vi "TRIGGER-completoN (SubVI).vi"(1 "Modalità":bool, 2 "isteresi":dbl, 3 "livello":dbl, 4 "Segnale B":dbl[](array[numeric])) -> (0 "eventi di trigger":i32[](array[numeric]))   [LabVIEW 2018]
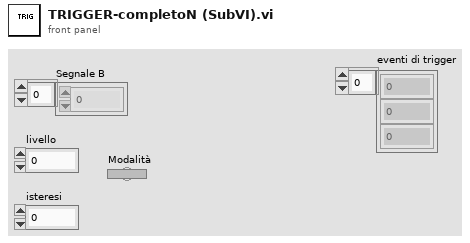
[diagram p1: front panel]
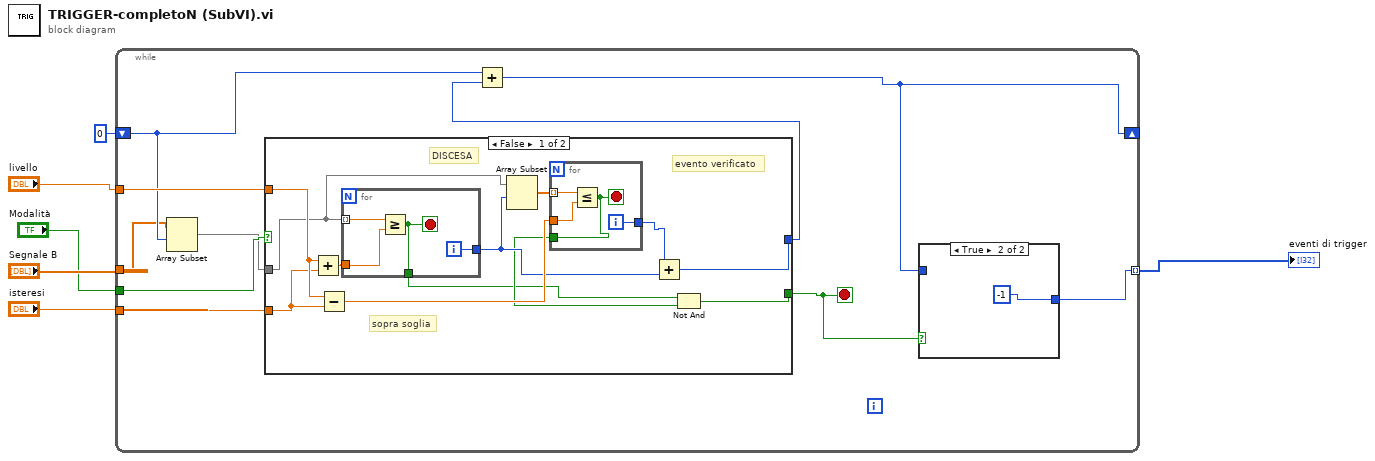
[diagram p0: block diagram]
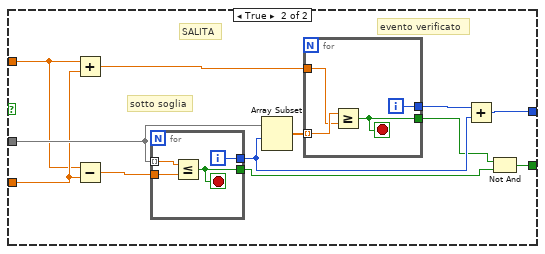
[diagram p3: hidden frame]
diagram:
  n1 = while {
    tunnel: "Segnale B" -> [w9]
    tunnel: "isteresi" -> [w16]
    tunnel: "livello" -> [w15]
    tunnel: [w11] -> w1 mode=indexing
    shift-right: [w8] -> _
    shift-left: 0 -> [w13]
    tunnel: "Modalità" -> [w12]
    stop <- w7 stop-if-true
    n2 = Array Subset(array=w9, index=w13) -> (w10:dbl[])  [unwired: 1 in]
    n3 = case shown="False" w12 {
      tunnel: w10 -> [w22 w49]
      tunnel: w16 -> [w24 w46]
      tunnel: w15 -> [w25 w45]
      tunnel: [w27 w42] -> w14
      tunnel: [w19 w41] -> w7
      frame False {
        # "evento verificato"
        # "sopra soglia"
        # "DISCESA"
        n4 = Add(x=w25, y=w24) -> (x+y=w26:dbl)
        n5 = Subtract(x=w25, y=w24) -> (x-y=w30:dbl)
        n6 = for {
          tunnel: [w38] -> w28
          tunnel: [w37] -> w20
          tunnel: w22 -> [w36] mode=indexing
          tunnel: w26 -> [w35]
          i -> [w38]
          stop <- w37 stop-if-true
          n7 = Greater Or Equal?(x=w36, y=w35) -> (x >= y?=w37:bool)
        }
        n8 = Array Subset(array=w22, index=w28) -> (w23:dbl[])  [unwired: 1 in]
        n9 = for {
          tunnel: w30 -> [w34]
          tunnel: [w33] -> w29
          tunnel: [w32] -> w21
          tunnel: w23 -> [w31] mode=indexing
          i -> [w33]
          stop <- w32 stop-if-true
          n10 = Less Or Equal?(x=w31, y=w34) -> (x <= y?=w32:bool)
        }
        n11 = Add(x=w29, y=w28) -> (x+y=w27:i32)
        n12 = Not And(1:w21, 2:w20) -> (0:w19:bool)
      }
      frame True {
        # "evento verificato"
        # "sotto soglia"
        # "SALITA"
        n13 = Add(x=w45, y=w46) -> (x+y=w47:dbl)
        n14 = Subtract(x=w45, y=w46) -> (x-y=w44:dbl)
        n15 = for {
          tunnel: w49 -> [w56] mode=indexing
          tunnel: w44 -> [w57]
          tunnel: [w58] -> w50
          tunnel: [w55] -> w40
          i -> [w58]
          stop <- w55 stop-if-true
          n16 = Less Or Equal?(x=w56, y=w57) -> (x <= y?=w55:bool)
        }
        n17 = Array Subset(array=w49, index=w50) -> (w48:dbl[])  [unwired: 1 in]
        n18 = for {
          tunnel: w48 -> [w53] mode=indexing
          tunnel: w47 -> [w52]
          tunnel: [w54] -> w43
          tunnel: [w51] -> w39
          i -> [w54]
          stop <- w51 stop-if-true
          n19 = Greater Or Equal?(x=w53, y=w52) -> (x >= y?=w51:bool)
        }
        n20 = Add(x=w43, y=w50) -> (x+y=w42:i32)
        n21 = Not And(1:w40, 2:w39) -> (0:w41:bool)
      }
    }
    n22 = Add(x=w13, y=w14) -> (x+y=w8:i32)
    n23 = case shown="True" w7 {
      tunnel: [w17 -1] -> w11
      tunnel: w8 -> [w17 _]
      frame False {
      }
      frame True {
      }
    }
  }
  "eventi di trigger" <- w1
